vi "Revision Query.vi"(8 "error in (no error)":errorcluster, 11 "VISA resource name":refnum<visa-resource-name>) -> (0 "error out":errorcluster, 1 "Instrument Firmware Revision":string, 2 "Instrument Driver Revision":string, 3 "VISA resource name out":refnum<visa-resource-name>, 4 "Instrument Serial Number":string)   [LabVIEW 2012, in "Ocean Optics 2000 4000.lvlib"]
doc: "Queries the current instrument firmware revision and instrument driver revision.\n\nRefer to the Readme file for detailed driver information including modification history."
uses:
  Ocean Optics 2000 4000.lvlib
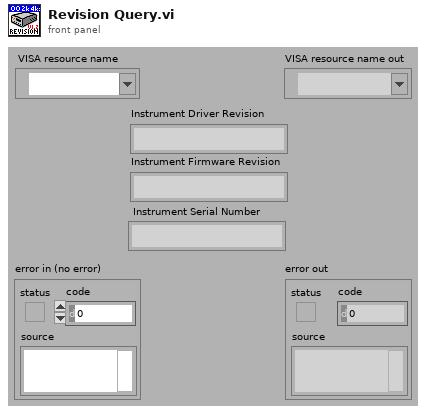
[diagram p1: front panel]
types:
  T1 = enum32{"invalid app kind", "Development System", "Run Time System", "Student Edition", "Embedded LabVIEW", "Evaluation", "Custom"}
  T2 = cluster{"Major":u16, "Minor":u16, "Fix":u16, "Build":u16}
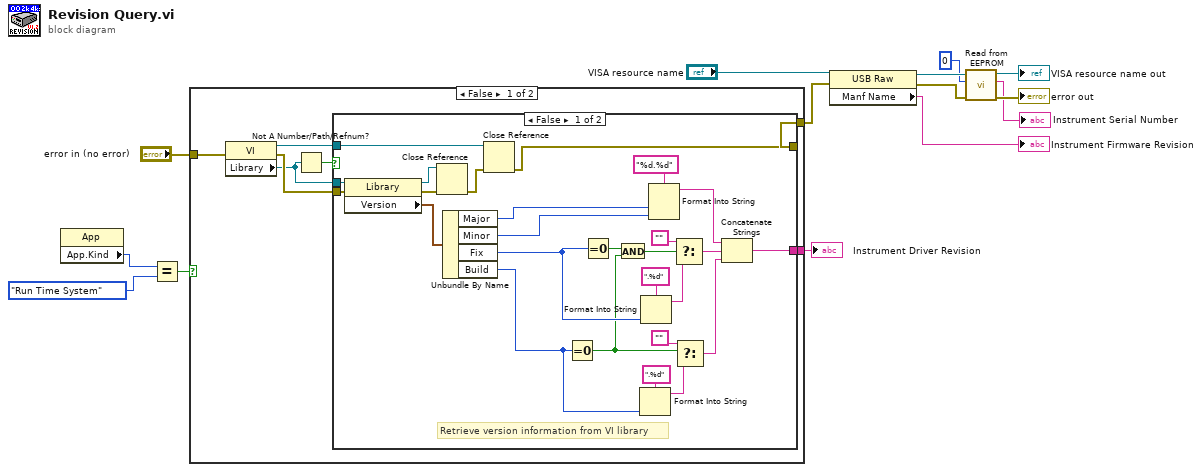
[diagram p0: block diagram]
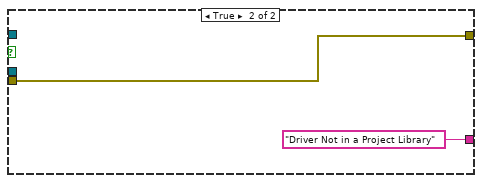
[diagram p2: hidden frame]
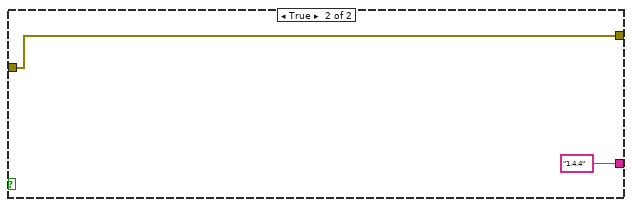
[diagram p3: hidden frame]
diagram:
  n1 = property class="App"() -> ("App.Kind"=w11:T1)  [unwired: 2 in, 2 out]
  n2 = Equal?(x=w11, y=T1."Run Time System" ("Application:Kind")) -> (x = y?=w12:bool)
  n3 = case shown="False" w12 {
    tunnel: [w17 "1.4.4"] -> w14
    tunnel: "error in (no error)" -> [w16 w50]
    tunnel: [w15 w50] -> w8
    frame False {
      n4 = property class="VI"(error in=w16) -> (reference out=w21:refnum<vi>, error out=w20:errorcluster, "Library"=w19:refnum<vi>)  [unwired: 1 in]
      n5 = Not A Number/Path/Refnum?(number/path/refnum=w19) -> (NaN/Path/Refnum?=w18:bool)
      n6 = case shown="False" w18 {
        tunnel: w21 -> [w44 _]
        tunnel: w20 -> [w29 w49]
        tunnel: [w24 w49] -> w15
        tunnel: [w23 "Driver Not in a Project Library"] -> w17
        tunnel: w19 -> [w22 _]
        frame False {
          # "Retrieve version information from VI library"
          n7 = property class="Library"(reference=w22, error in=w29) -> (reference out=w46:refnum<vi>, error out=w47:errorcluster, "Version"=w43:T2)
          n8 = Close Reference(reference=w46, error in (no error)=w47) -> (error out=w45:errorcluster)
          n9 = Unbundle By Name(w43) -> ("Major"=w32:u16, "Minor"=w31:u16, "Fix"=w28:u16, "Build"=w30:u16)
          n10 = Close Reference(reference=w44, error in (no error)=w45) -> (error out=w24:errorcluster)
          n11 = Equal To 0?(x=w30) -> (x = 0?=w26:bool)
          n12 = Equal To 0?(x=w28) -> (x = 0?=w27:bool)
          n13 = And(x=w27, y=w26) -> (x .and. y?=w25:bool)
          n14 = Format Into String(format string=".%d", w30) -> (resulting string=w36:string)  [unwired: 2 in, 1 out]
          n15 = Format Into String(format string=".%d", w28) -> (resulting string=w40:string)  [unwired: 2 in, 1 out]
          n16 = Format Into String(format string="%d.%d", w32, w31) -> (resulting string=w38:string)  [unwired: 2 in, 1 out]
          n17 = Select(t="", s=w25, f=w40) -> (s? t:f=w37:string)
          n18 = Select(t="", s=w26, f=w36) -> (s? t:f=w33:string)
          n19 = Concatenate Strings(w38, w37, w33) -> (w23:string)
        }
        frame True {
        }
      }
    }
    frame True {
    }
  }
  "Instrument Driver Revision" <- w14
  n20 = property class="USB Raw"(reference="VISA resource name", error in=w8) -> (reference out=w6:refnum<visa-resource-name>, error out=w4:errorcluster, "Manf Name"=→"Instrument Firmware Revision":string)
  n21 = call "Read from EEPROM.vi"("error in (no error)"=w4, "EEPROM Index"=u8 0, "VISA resource name"=w6) -> ("error out"=→"error out":errorcluster, "ASCII Data"=→"Instrument Serial Number":string, "VISA resource name out"=→"VISA resource name out":refnum<visa-resource-name>)  [unwired: 6 out]
